vi "ReadM1PositionPID.vi"(0 "VISA Refnum in":refnum<visa-resource-name>, 5 "Address":u8, 11 "error in (no error)":errorcluster) -> (1 "Kp":u32, 2 "Ki":u32, 3 "Kd":u32, 4 "VISA Refnum out":refnum<visa-resource-name>, 6 "Valid":bool, 10 "KiMax":u32, 12 "MaxPos":u32, 13 "MinPos":u32, 14 "Deadzone":u32, 15 "error out":errorcluster)   [LabVIEW 2015, in "Ion Motion Roboclaw.lvlib"]
uses:
  <instrlib>/Ion Motion Roboclaw/Ion Motion Roboclaw.lvlib
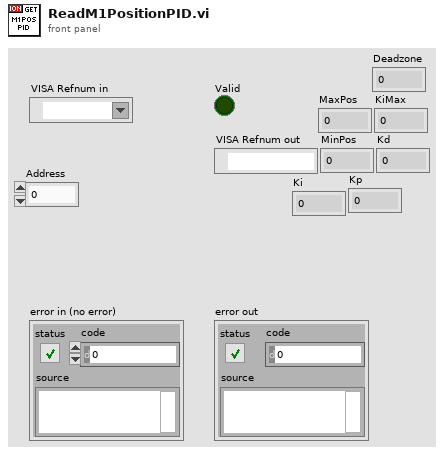
[diagram p1: front panel]
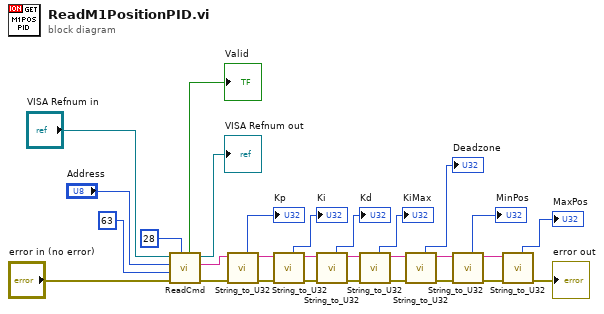
[diagram p0: block diagram]
diagram:
  n1 = call <instrlib>:"ReadCmd.vi"("Read Count"=u32 28, "error in (no error)"="error in (no error)", "Cmd"=u8 63, "Address"="Address", "VISA Refnum in"="VISA Refnum in") -> ("error out"=w7:errorcluster, "Output"=w8:string, "VISA Refnum out"=→"VISA Refnum out":refnum<visa-resource-name>, "Valid"=→"Valid":bool)  [unwired: 3 in]
  n2 = call <instrlib>:"String_to_U32.vi"("error in (no error)"=w7, "String"=w8) -> ("error out"=w23:errorcluster, "rest of the binary string"=w29:string, "number"=→"Kp":u32)  [unwired: 5 in]
  n3 = call <instrlib>:"String_to_U32.vi"("error in (no error)"=w23, "String"=w29) -> ("error out"=w22:errorcluster, "rest of the binary string"=w28:string, "number"=→"Ki":u32)  [unwired: 5 in]
  n4 = call <instrlib>:"String_to_U32.vi"("error in (no error)"=w22, "String"=w28) -> ("error out"=w21:errorcluster, "rest of the binary string"=w27:string, "number"=→"Kd":u32)  [unwired: 5 in]
  n5 = call <instrlib>:"String_to_U32.vi"("error in (no error)"=w21, "String"=w27) -> ("error out"=w20:errorcluster, "rest of the binary string"=w26:string, "number"=→"KiMax":u32)  [unwired: 5 in]
  n6 = call <instrlib>:"String_to_U32.vi"("error in (no error)"=w20, "String"=w26) -> ("error out"=w19:errorcluster, "rest of the binary string"=w25:string, "number"=→"Deadzone":u32)  [unwired: 5 in]
  n7 = call <instrlib>:"String_to_U32.vi"("error in (no error)"=w19, "String"=w25) -> ("error out"=w18:errorcluster, "rest of the binary string"=w24:string, "number"=→"MinPos":u32)  [unwired: 5 in]
  n8 = call <instrlib>:"String_to_U32.vi"("error in (no error)"=w18, "String"=w24) -> ("error out"=→"error out":errorcluster, "number"=→"MaxPos":u32)  [unwired: 5 in, 1 out]
